vi "sample_ts_tree.vi"() -> ()   [LabVIEW 2015]
uses:
  controls/marquardt-tree.ctl
  ts-data.ctl
panel:
  out "Active Item:Indent Level":i32
  out "Active Item:Tag":string
  out "Value":string
  out "Active Cell:Active Column Number":i32
  out "Active Item:Row Number":i32
  out "Active Cell:String":string
  in  "stop":bool
  in  "Tree":T1
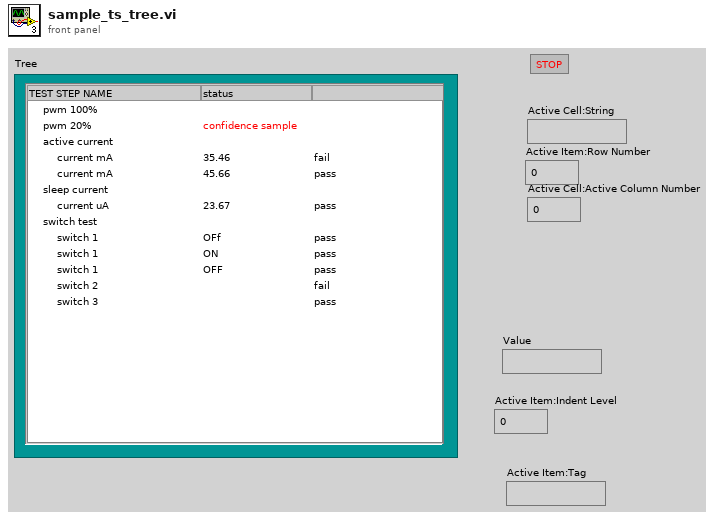
[diagram p1: front panel]
types:
  T1 = typedef "marquardt-tree.ctl" = string
  T2 = typedef "ts-data.ctl" = cluster{"ts.tag":string, "ts.desc":string, "ts.method":string}
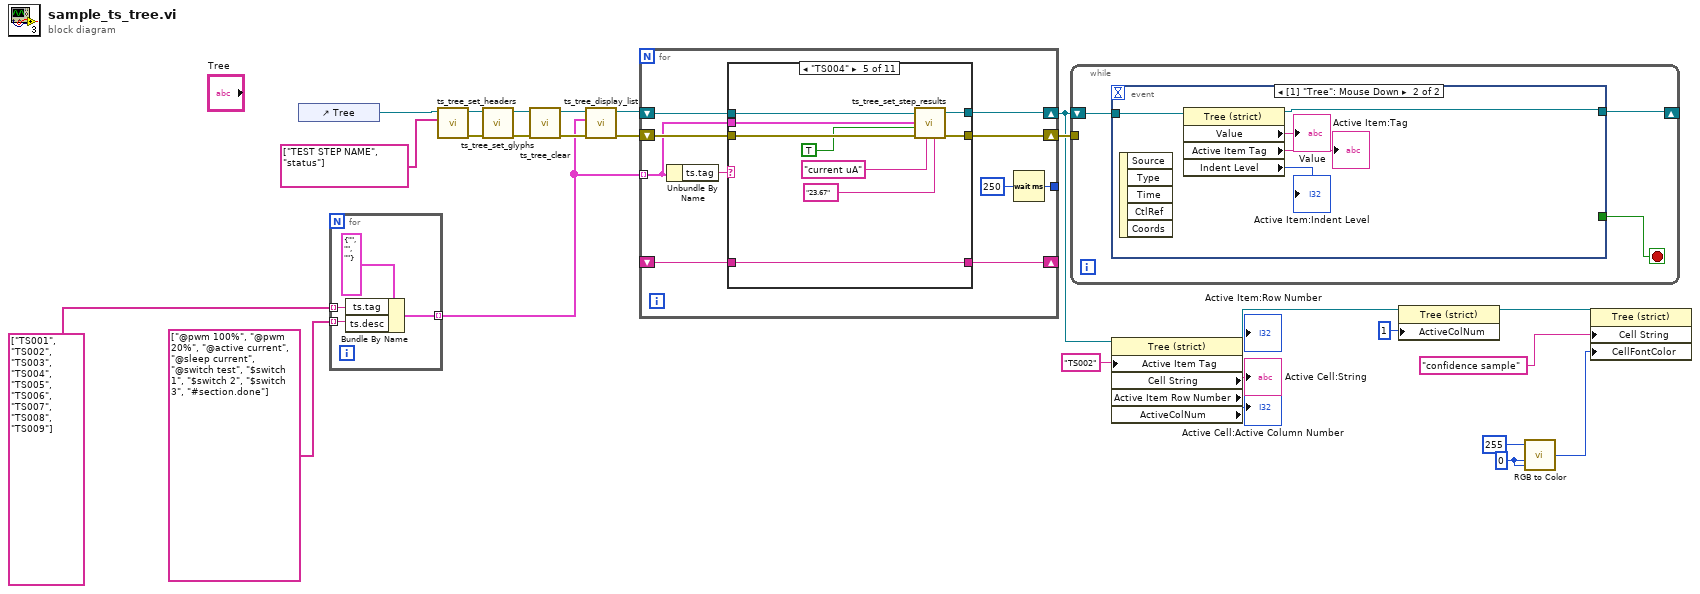
[diagram p0: block diagram]
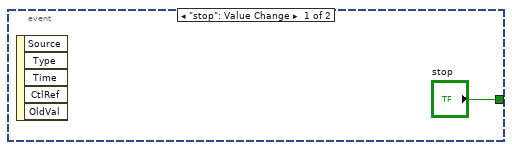
[diagram p2: hidden frame]
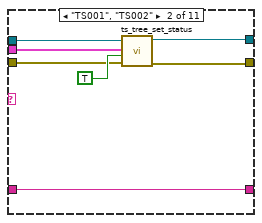
[diagram p4: hidden frame]
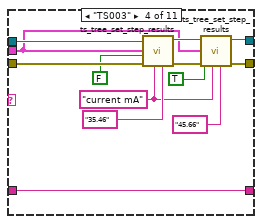
[diagram p6: hidden frame]
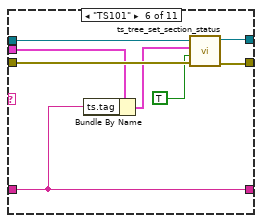
[diagram p7: hidden frame]
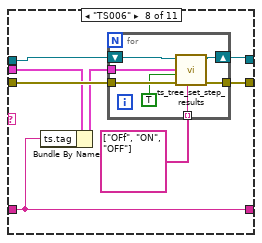
[diagram p9: hidden frame]
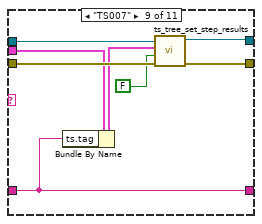
[diagram p10: hidden frame]
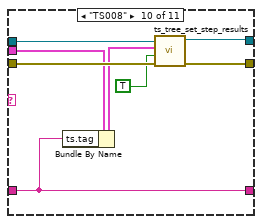
[diagram p11: hidden frame]
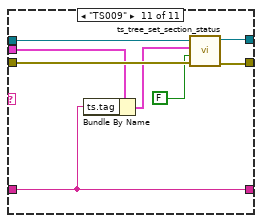
[diagram p12: hidden frame]
diagram:
  w4 = u8 0 ("G")
  n1 = control-ref of="Tree"() -> (w22:refnum<vi>)
  n2 = for {
    tunnel: string[] ["TS001", "TS002", "TS003", "TS004", "TS005", "TS006", "TS007", "TS008", "TS009"] -> [w28] mode=indexing
    tunnel: string[] ["@pwm 100%", "@pwm 20%", "@active current", "@sleep current", "@switch test", "$switch 1", "$switch 2", "$switch 3", "#section.done"] -> [w27] mode=indexing
    tunnel: [w26] -> w19 mode=indexing
    n3 = Bundle By Name(cluster=T2 {"ts.tag"="", "ts.desc"="", "ts.method"=""} ("ts.data"), "ts.tag"=w28, "ts.desc"=w27) -> (w26:T2)
  }
  n4 = call "ts_tree_set_headers.vi"("headers"=string[] ["TEST STEP NAME", "status"], "Tree.in"=w22) -> ("error out"=w13:errorcluster, "Tree.out"=w12:refnum<vi>)  [unwired: 8 in]
  n5 = call "ts_tree_set_glyphs.vi"("error in"=w13, "Tree.in"=w12) -> ("error out"=w15:errorcluster, "Tree.out"=w14:refnum<vi>)  [unwired: 8 in]
  n6 = call "ts_tree_clear.vi"("error in (no error)"=w15, "Tree.in"=w14) -> ("error out"=w20:errorcluster, "Tree.out"=w21:refnum<vi>)  [unwired: 8 in]
  n7 = call "ts_tree_display_list.vi"("error in (no error)"=w20, "ts.list"=w19, "Tree.in"=w21) -> ("error out"=w17:errorcluster, "Tree.out"=w18:refnum<vi>)  [unwired: 7 in]
  n8 = for {
    tunnel: w19 -> [w35] mode=indexing
    shift-right: [w37] -> w1
    shift-left: w18 -> [w38]
    shift-right: [w34] -> w16
    shift-left: w17 -> [w36]
    tunnel: [w33] -> _
    shift-right: [w31] -> _
    shift-left: _ -> [w30]
    n9 = Unbundle By Name(w35) -> ("ts.tag"=w39:string)
    n10 = case shown="\"TS004\"" w39 {
      selector: w39 -> [_ _ w52 _ _ _ w83 _ _ _ _]
      tunnel: w38 -> [w42 w49 w50 w65 w74 w82 w85 w91 w106 w114 w124]
      tunnel: [w42 w48 w50 w55 w73 w81 w85 w89 w105 w113 w123] -> w37
      tunnel: w36 -> [w41 w46 w51 w64 w72 w80 w84 w93 w108 w116 w122]
      tunnel: w35 -> [_ w45 _ w53 w66 w77 _ w92 w103 w111 w119]
      tunnel: [w41 w44 w51 w56 w71 w79 w84 w88 w107 w115 w121] -> w34
      tunnel: [w40 w43 w52 w54 w67 w75 w83 w86 w101 w109 w117] -> w31
      tunnel: w30 -> [w40 w43 _ w54 w67 w75 _ w86 w101 w109 w117]
      frame "False", Default {
      }
      frame "TS001", "TS002" {
        n11 = call "ts_tree_set_status.vi"("error in (no error)"=w46, "ts.status"=TRUE, "ts.data"=w45, "Tree.in"=w49) -> ("error out"=w44:errorcluster, "Tree.out"=w48:refnum<vi>)  [unwired: 6 in]
      }
      frame "TS100" {
      }
      frame "TS003" {
        w58 = "current mA"
        n12 = call "ts_tree_set_step_results.vi"("results.data"="35.46", "results.txt"=w58, "error in (no error)"=w64, "ts.status"=FALSE, "ts.data"=w53, "Tree.in"=w65) -> ("error out"=w60:errorcluster, "Tree.out"=w61:refnum<vi>)  [unwired: 4 in]
        n13 = call "ts_tree_set_step_results.vi"("results.data"="45.66", "results.txt"=w58, "error in (no error)"=w60, "ts.status"=TRUE, "ts.data"=w53, "Tree.in"=w61) -> ("error out"=w56:errorcluster, "Tree.out"=w55:refnum<vi>)  [unwired: 4 in]
      }
      frame "TS004" {
        n14 = call "ts_tree_set_step_results.vi"("results.data"="23.67", "results.txt"="current uA", "error in (no error)"=w72, "ts.status"=TRUE, "ts.data"=w66, "Tree.in"=w74) -> ("error out"=w71:errorcluster, "Tree.out"=w73:refnum<vi>)  [unwired: 4 in]
      }
      frame "TS101" {
        n15 = Bundle By Name(cluster=w77, "ts.tag"=w75) -> (w76:T2)
        n16 = call "ts_tree_set_section_status.vi"("error in (no error)"=w80, "ts.status"=TRUE, "ts.data"=w76, "Tree.in"=w82) -> ("error out"=w79:errorcluster, "Tree.out"=w81:refnum<vi>)  [unwired: 6 in]
      }
      frame "TS005" {
      }
      frame "TS006" {
        n17 = Bundle By Name(cluster=w92, "ts.tag"=w86) -> (w87:T2)
        n18 = for {
          tunnel: w93 -> [w100]
          tunnel: w87 -> [w99]
          tunnel: [w96] -> w88
          shift-right: [w97] -> w89
          shift-left: w91 -> [w98]
          tunnel: string[] ["OFf", "ON", "OFF"] -> [w94] mode=indexing
          n19 = call "ts_tree_set_step_results.vi"("results.txt"=w94, "error in (no error)"=w100, "ts.status"=TRUE, "ts.data"=w99, "Tree.in"=w98) -> ("error out"=w96:errorcluster, "Tree.out"=w97:refnum<vi>)  [unwired: 5 in]
        }
      }
      frame "TS007" {
        n20 = Bundle By Name(cluster=w103, "ts.tag"=w101) -> (w102:T2)
        n21 = call "ts_tree_set_step_results.vi"("error in (no error)"=w108, "ts.status"=FALSE, "ts.data"=w102, "Tree.in"=w106) -> ("error out"=w107:errorcluster, "Tree.out"=w105:refnum<vi>)  [unwired: 6 in]
      }
      frame "TS008" {
        n22 = Bundle By Name(cluster=w111, "ts.tag"=w109) -> (w110:T2)
        n23 = call "ts_tree_set_step_results.vi"("error in (no error)"=w116, "ts.status"=TRUE, "ts.data"=w110, "Tree.in"=w114) -> ("error out"=w115:errorcluster, "Tree.out"=w113:refnum<vi>)  [unwired: 6 in]
      }
      frame "TS009" {
        n24 = Bundle By Name(cluster=w119, "ts.tag"=w117) -> (w118:T2)
        n25 = call "ts_tree_set_section_status.vi"("error in (no error)"=w122, "ts.status"=FALSE, "ts.data"=w118, "Tree.in"=w124) -> ("error out"=w121:errorcluster, "Tree.out"=w123:refnum<vi>)  [unwired: 6 in]
      }
    }
    n26 = Wait (ms)(milliseconds to wait=u32 250) -> (millisecond timer value=w33:u32)
  }
  n27 = while {
    tunnel: w16 -> [_]
    shift-right: [w125] -> _
    shift-left: w1 -> [w126]
    stop <- w127 stop-if-true
    n28 = event shown="[1] \"Tree\": Mouse Down" {
      selector: _ -> [_ _]
      dyn-events: _ -> [_ _]
      timeout: _ -> [_ _]
      tunnel: ["stop" _] -> w127
      tunnel: w126 -> [_ w133]
      tunnel: [_ w129] -> w125
      event "stop": Value Change {
        n29 = event-data() -> ()  [unwired: 1 in, 5 out]
      }
      event Mouse Down {
        n30 = event-data() -> ()  [unwired: 1 in, 5 out]
        n31 = property class="Tree (strict)"(reference=w133) -> (reference out=w129:refnum<vi>, "Value"=→"Value":string, "Active Item Tag"=→"Active Item:Tag":string, "Indent Level"=→"Active Item:Indent Level":i32)  [unwired: 1 in, 1 out]
      }
    }
  }
  n32 = property class="Tree (strict)" props=["Active Item Tag", "Cell String", "Active Item Row Number", "ActiveColNum"](reference=w1, "Active Item Tag"="TS002" ("Active Item:Tag")) -> (reference out=w9:refnum<vi>, "Cell String"=→"Active Cell:String":string, "ActiveColNum"=→"Active Cell:Active Column Number":i32)  [unwired: 1 in, 2 out]
  n33 = property class="Tree (strict)"(reference=w9, "ActiveColNum"=1 ("Active Cell:Active Column Number")) -> (reference out=w7:refnum<vi>)  [unwired: 1 in, 1 out]
  n34 = call <vilib>:"RGB to Color.vi"("B"=w4, "G"=w4, "R"=u8 255) -> ("Color"=w3:u32)
  n35 = property class="Tree (strict)"(reference=w7, "Cell String"="confidence sample" ("Active Cell:String"), "CellFontColor"=w3) -> ()  [unwired: 1 in, 2 out]
